vi "Parse Notification.vi"(8 "error in (no error)":errorcluster, 10 "Response body":string) -> (0 "error out":errorcluster, 3 "Notification Configuration":T1)   [LabVIEW 2015, in "NI_AWS_S3.lvlib"]
uses:
  NI_AWS_S3.lvlib
  Notification Configuration.ctl
  Topic Configuration.ctl
  Event.ctl
  Core/HTTP Request/Name Value Pair.ctl
  Cloud Function Configuration.ctl
  Queue Configuration.ctl
  Core/HTTP Request/HTTP Request.lvclass
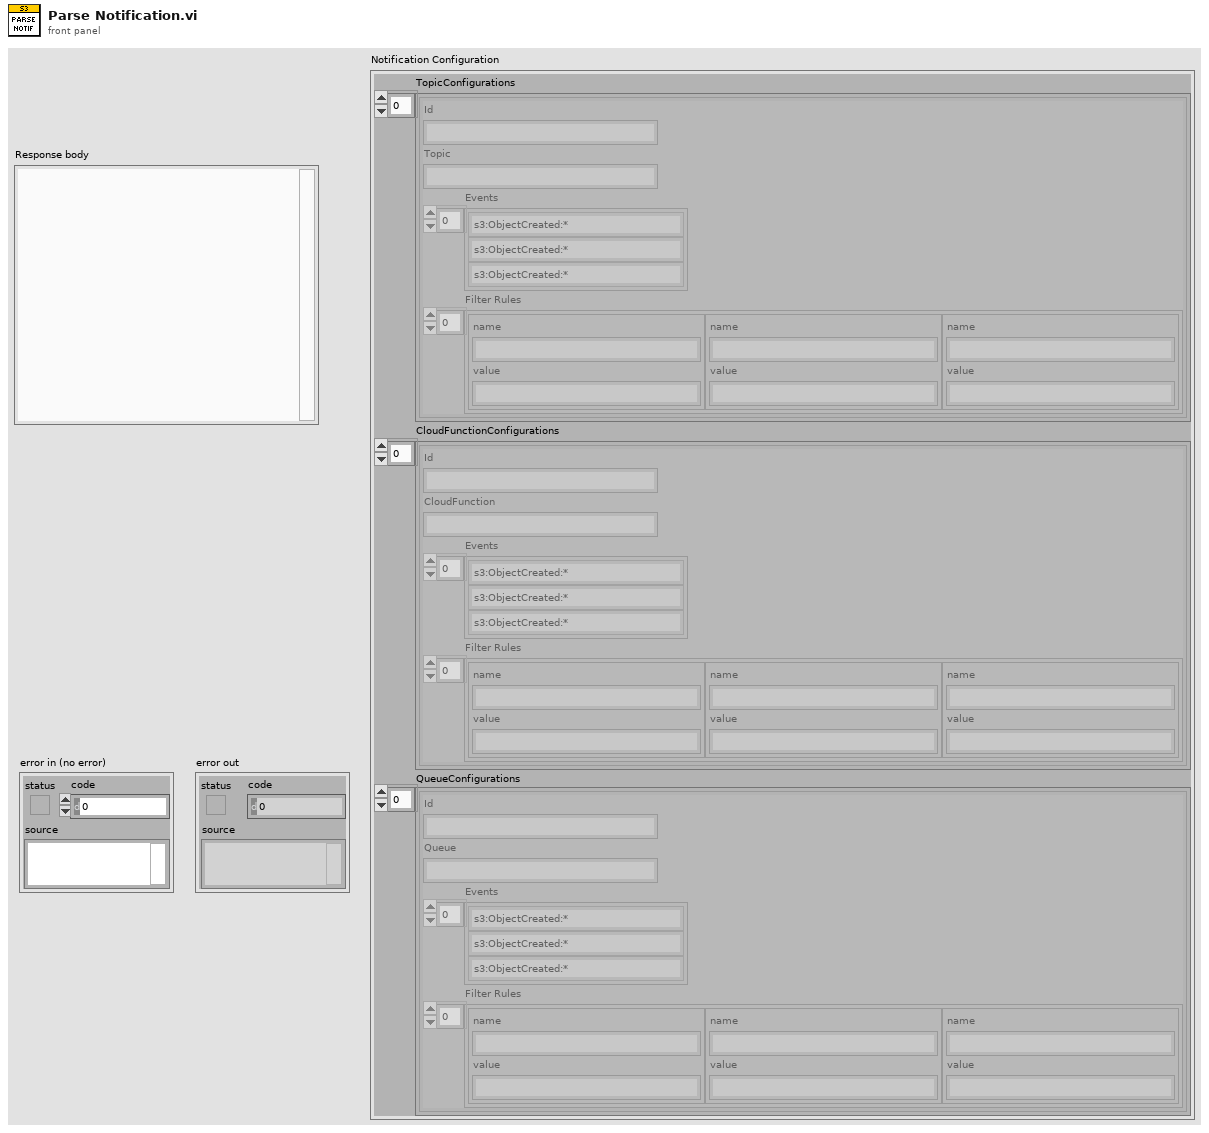
[diagram p1: front panel]
types:
  T1 = typedef "NI_AWS_S3.lvlib/Notification Configuration.ctl" = cluster{"TopicConfigurations":T2[], "CloudFunctionConfigurations":T5[], "QueueConfigurations":T6[]}
  T2 = typedef "NI_AWS_S3.lvlib/Topic Configuration.ctl" = cluster{"Id":string, "Topic":string, "Events":T3[], "Filter Rules":T4[]}
  T3 = typedef "NI_AWS_S3.lvlib/Event.ctl" = enum16{"s3:ObjectCreated:*", "s3:ObjectCreated:Put", "s3:ObjectCreated:Post", "s3:ObjectCreated:Copy", "s3:ObjectCreated:CompleteMultipartUpload", "s3:ObjectRemoved:*", "s3:ObjectRemoved:Delete", "s3:ObjectRemoved:DeleteMarkerCreated", "s3:ReducedRedundancyLostObject"}
  T4 = typedef "NI_AWS_Core.lvlib/HTTP Request.lvclass/Name Value Pair.ctl" = cluster{"name":string, "value":string}
  T5 = typedef "NI_AWS_S3.lvlib/Cloud Function Configuration.ctl" = cluster{"Id":string, "CloudFunction":string, "Events":T3[], "Filter Rules":T4[]}
  T6 = typedef "NI_AWS_S3.lvlib/Queue Configuration.ctl" = cluster{"Id":string, "Queue":string, "Events":T3[], "Filter Rules":T4[]}
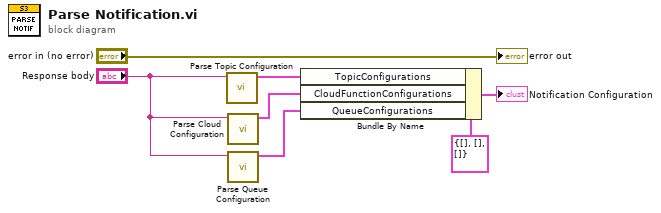
[diagram p0: block diagram]
diagram:
  n1 = call "Parse Topic Configuration.vi"("Response body"="Response body") -> ("Topic Configurations"=w3:T2[])  [unwired: 10 in]
  n2 = call "Parse Cloud Configuration.vi"("Response body"="Response body") -> ("Cloud Function Configurations"=w5:T5[])  [unwired: 10 in]
  n3 = call "Parse Queue Configuration.vi"("Response body"="Response body") -> ("Queue Configurations"=w1:T6[])  [unwired: 10 in]
  n4 = Bundle By Name(cluster=T1 {"TopicConfigurations"=[], "CloudFunctionConfigurations"=[], "QueueConfigurations"=[]} ("NotificationConfiguration"), "TopicConfigurations"=w3, "CloudFunctionConfigurations"=w5, "QueueConfigurations"=w1) -> (→"Notification Configuration":T1)
  "error out" <- "error in (no error)"
